vi "PH_gentec_M-Link.set Trigger Source.vi"(0 "i ref in":refnum<vi>, 2 "VISA resource in":refnum<visa-resource-name>, 5 "error in":errorcluster) -> (14 "i ref out":refnum<vi>, 16 "VISA resource out":refnum<visa-resource-name>, 17 "Error":bool, 19 "error out":errorcluster)   [LabVIEW 2014, in "PH_gentec_M-Link.lvlib"]
doc: "This VI writes wanted Settings to the Device and checks the result."
uses:
  PH_gentec_M-Link.lvlib
  non_GPL/instr.lib/gentec-M-LINK/gentec-M-Link - Driver.lvlib
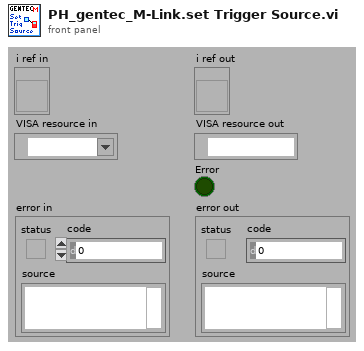
[diagram p1: front panel]
types:
  T1 = typedef "PH_gentec_M-Link.lvlib/PH_gentec_M-Link.i attribute.ctl" = cluster{"GUI References":cluster{"Wanted Head Settings":refnum<vi>, "Current Head Settings":refnum<vi>, "Set Auto Range":refnum<vi>, "Trigger Polarity":refnum<vi>, "Trigger Source":refnum<vi>, "Waveform Averages":refnum<vi>, "Continuous":refnum<vi>, "get one Value":refnum<vi>}, "Wanted Head Settings":T2, "Current Head Settings":T2}
  T2 = typedef "PH_gentec_M-Link.lvlib/PH_gentec_M-Link.Head Settings.ctl" = cluster{"Measurement Mode":T3, "Enable Anticipation":bool, "Set Auto Range":bool, "Block Signal":bool, "Set Head Attenuator":bool, "Enable SSE":bool, "Trigger Polarity":T4, "Trigger Source":T5, "Waveform Averages":T6, "Set Zero":i32, "Current Measurement":i32, "Start Data Flow":bool}
  T3 = typedef "gentec-M-Link - Driver.lvlib/gentec-M-Link.Measurement Mode.ctl" = u16
  T4 = typedef "gentec-M-Link - Driver.lvlib/gentec-M-Link.Trigger Polarity.ctl" = u16
  T5 = typedef "gentec-M-Link - Driver.lvlib/gentec-M-Link.Trigger Source.ctl" = u16
  T6 = typedef "gentec-M-Link - Driver.lvlib/gentec-M-Link.Waveform Averages.ctl" = u16
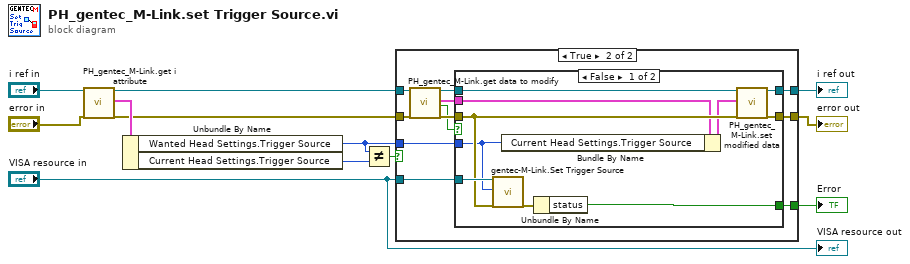
[diagram p0: block diagram]
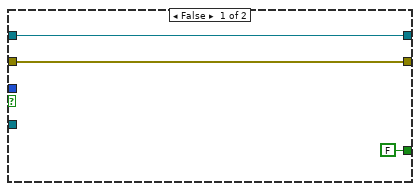
[diagram p2: hidden frame]
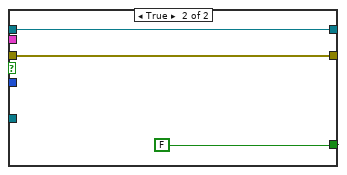
[diagram p3: hidden frame]
diagram:
  n1 = call "PH_gentec_M-Link.get i attribute.vi"("i ref in"="i ref in", "error in (no error)"="error in") -> ("i ref out"=w6:refnum<vi>, "i attribute"=w9:T1, "error out"=w8:errorcluster)  [unwired: 15 in]
  n2 = Unbundle By Name(w9) -> ("Wanted Head Settings.Trigger Source"=w10:T5, "Current Head Settings.Trigger Source"=w1:T5)
  n3 = Not Equal?(x=w10, y=w1) -> (x != y?=w2:bool)
  n4 = case shown="True" w2 {
    tunnel: [w13 w26] -> w12
    tunnel: [w14 w25] -> w11
    tunnel: w10 -> [_ w24]
    tunnel: w8 -> [w13 w19]
    tunnel: w6 -> [w14 w18]
    tunnel: "VISA resource in" -> [_ w17]
    tunnel: [FALSE w16] -> w3
    frame False {
    }
    frame True {
      n5 = call "PH_gentec_M-Link.get data to modify.vi"("i ref in"=w18, "error in (no error)"=w19) -> ("i ref out"=w22:refnum<vi>, "i attribute"=w21:T1, "timed out"=w20:bool, "error out"=w23:errorcluster)  [unwired: 14 in]
      n6 = case shown="False" w20 {
        tunnel: w17 -> [w35 _]
        tunnel: [w32 w39] -> w25
        tunnel: [w31 w38] -> w26
        tunnel: w23 -> [w34 w38]
        tunnel: w22 -> [w36 w39]
        tunnel: w21 -> [w33 _]
        tunnel: w24 -> [w27 _]
        tunnel: [w29 FALSE] -> w16
        frame False {
          n7 = call "gentec-M-Link.Set Trigger Source.vi"("VISA resource In"=w35, "Trigger Source"=w27, "error in (no error)"=w34) -> ("error out"=w28:errorcluster)  [unwired: 15 in, 1 out]
          n8 = Bundle By Name(cluster=w33, "Current Head Settings.Trigger Source"=w27) -> (w30:T1)
          n9 = Unbundle By Name(w28) -> ("status"=w29:bool)
          n10 = call "PH_gentec_M-Link.set modified data.vi"("i ref in"=w36, "i attribute"=w30, "error in (no error)"=w34) -> ("i ref out"=w32:refnum<vi>, "error out"=w31:errorcluster)  [unwired: 15 in]
        }
        frame True {
        }
      }
    }
  }
  "error out" <- w12
  "i ref out" <- w11
  "Error" <- w3
  "VISA resource out" <- "VISA resource in"
